vi "OPC.vi"(8 "error in (no error)":errorcluster, 11 "E5071C in":refnum<class "E5071C.lvclass">) -> (0 "error out":errorcluster, 3 "E5071C out":refnum<class "E5071C.lvclass">)   [LabVIEW 2020, in "E5071C.lvlib" / "E5071C.lvclass"]
uses:
  E5071C.lvclass
  E5071C.lvclass/E5071C.ctl
panel:
  out "String":string
  in  "Number Of Bytes":i32=-1
  out "Returned Bytes":i32
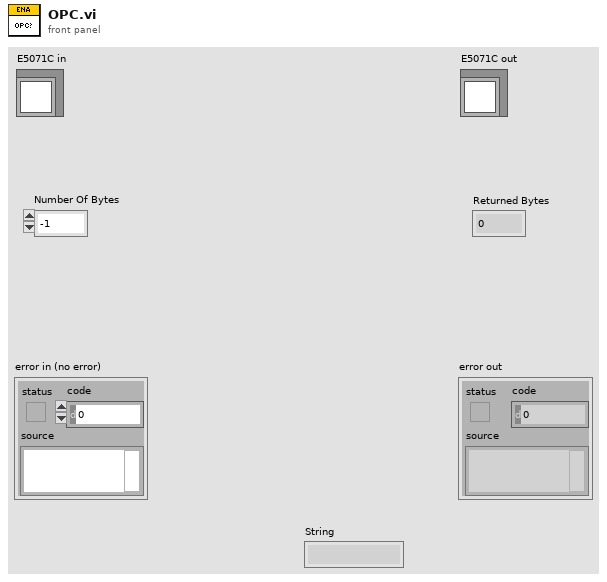
[diagram p1: front panel]
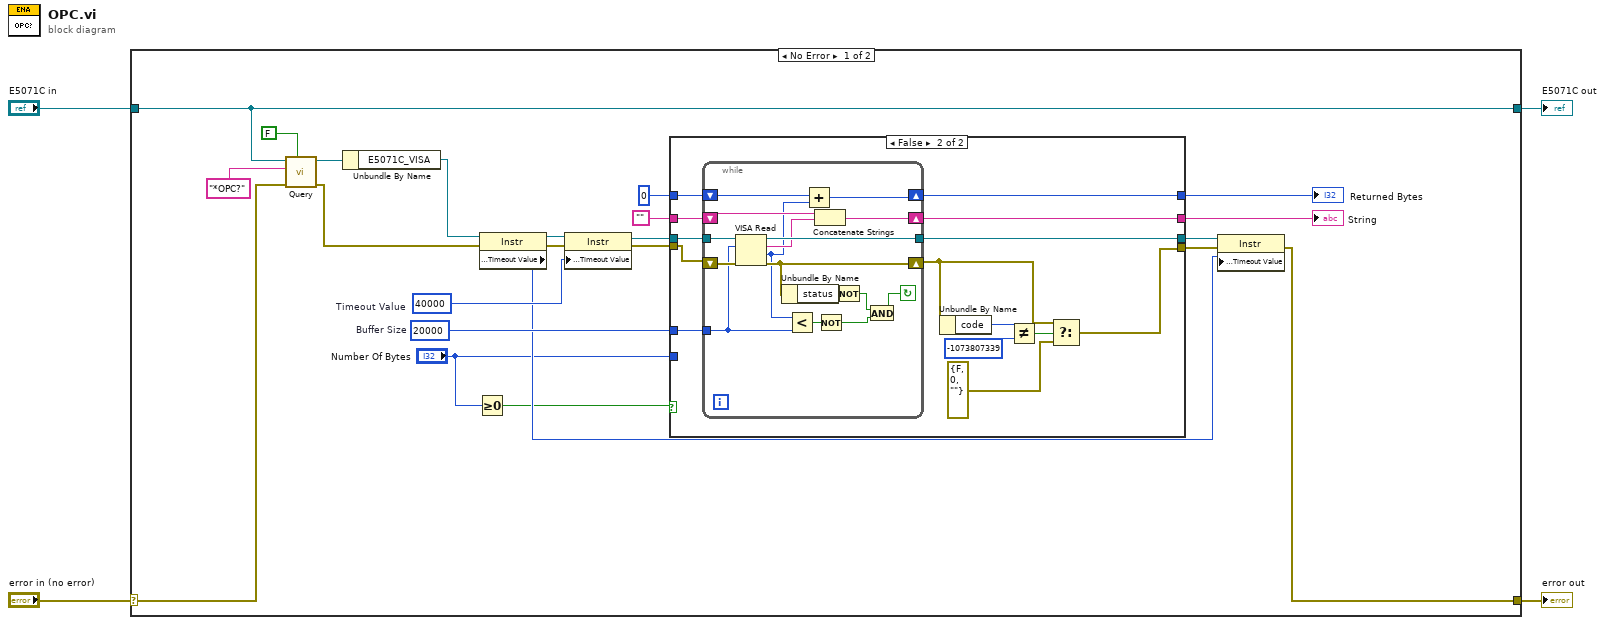
[diagram p0: block diagram]
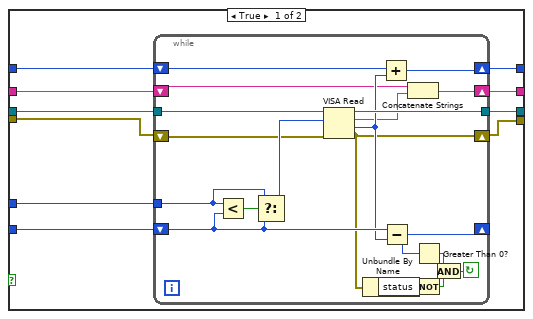
[diagram p2: hidden frame]
diagram:
  n1 = case shown="No Error" "error in (no error)" {
    selector: "error in (no error)" -> [w24 w88]
    tunnel: [w5 w88] -> w3
    tunnel: [w27 w87] -> w1
    tunnel: "E5071C in" -> [w27 w87]
    frame No Error {
      w15 = u32 40000  # Timeout Value
      w20 = u32 20000  # Buffer Size
      n2 = call "Query.vi"("Return"=FALSE, "error in (no error)"=w24, "Command"="*OPC?" ("write buffer"), "E5071C in"=w27) -> ("error out"=w6:errorcluster, "E5071C out"=w23:refnum<class "E5071C.lvclass">)  [unwired: 5 in, 1 out]
      n3 = Unbundle By Name(w23) -> ("E5071C_VISA"=w7:refnum<visa-resource-name>)
      n4 = Greater Or Equal To 0?(x="Number Of Bytes") -> (x >= 0?=w8:bool)
      n5 = property class="Instr"(reference=w7, error in=w6) -> (reference out=w17:refnum<visa-resource-name>, error out=w16:errorcluster, "General Settings:Timeout Value"=w10:u32)
      n6 = property class="Instr"(reference=w17, error in=w16, "General Settings:Timeout Value"=w15) -> (reference out=w13:refnum<visa-resource-name>, error out=w14:errorcluster)
      n7 = case shown="False" w8 {
        tunnel: "" -> [w37 w70]
        tunnel: [w36 w69] -> w21
        tunnel: w20 -> [w35 w68]
        tunnel: "Number Of Bytes" -> [w34 _]
        tunnel: u32 0 ("byte count (0)") -> [w33 w67]
        tunnel: [w32 w66] -> w18
        tunnel: w14 -> [w31 w65]
        tunnel: w13 -> [w30 w64]
        tunnel: [w29 w63] -> w12
        tunnel: [w28 w57] -> w11
        frame True {
          n8 = while {
            shift-left: w37 -> [w41]
            shift-right: [w42] -> w32
            tunnel: w35 -> [w50]
            shift-left: w33 -> [w48]
            shift-right: [w47] -> w36
            shift-left: w34 -> [w52]
            shift-right: [w51] -> _
            shift-left: w31 -> [w38]
            shift-right: [w39] -> w28
            tunnel: [w55] -> w29
            tunnel: w30 -> [w56]
            stop <- w43 continue-if-true
            n9 = Less?(x=w50, y=w52) -> (x < y?=w54:bool)
            n10 = Select(t=w50, s=w54, f=w52) -> (s? t:f=w53:u32)
            n11 = VISA Read(VISA resource name=w56, byte count=w53, error in (no error)=w38) -> (VISA resource name out=w55:refnum<visa-resource-name>, read buffer=w40:string, return count=w49:u32, error out=w39:errorcluster)
            n12 = Unbundle By Name(w39) -> ("status"=w45:bool)
            n13 = Add(x=w48, y=w49) -> (x+y=w47:u32)
            n14 = Subtract(x=w52, y=w49) -> (x-y=w51:u32)
            n15 = Concatenate Strings(w41, w40) -> (w42:string)
            n16 = Greater Than 0?(x=w51) -> (x > 0?=w46:bool)
            n17 = Not(x=w45) -> (.not. x?=w44:bool)
            n18 = And(x=w46, y=w44) -> (x .and. y?=w43:bool)
          }
        }
        frame False {
          n19 = while {
            shift-left: w70 -> [w80]
            shift-right: [w81] -> w66
            tunnel: w68 -> [w71]
            shift-left: w67 -> [w84]
            shift-right: [w83] -> w69
            shift-left: w65 -> [w77]
            shift-right: [w78] -> w59
            tunnel: [w85] -> w63
            tunnel: w64 -> [w86]
            stop <- w73 continue-if-true
            n20 = VISA Read(VISA resource name=w86, byte count=w71, error in (no error)=w77) -> (VISA resource name out=w85:refnum<visa-resource-name>, read buffer=w79:string, return count=w72:u32, error out=w78:errorcluster)
            n21 = Unbundle By Name(w78) -> ("status"=w82:bool)
            n22 = Less?(x=w72, y=w71) -> (x < y?=w76:bool)
            n23 = Add(x=w84, y=w72) -> (x+y=w83:u32)
            n24 = Concatenate Strings(w80, w79) -> (w81:string)
            n25 = Not(x=w76) -> (.not. x?=w75:bool)
            n26 = Not(x=w82) -> (.not. x?=w74:bool)
            n27 = And(x=w74, y=w75) -> (x .and. y?=w73:bool)
          }
          n28 = Unbundle By Name(w59) -> ("code"=w62:i32)
          n29 = Not Equal?(x=w62, y=-1073807339) -> (x != y?=w60:bool)
          n30 = Select(t=w59, s=w60, f=errorcluster {"status"=FALSE, "code"=0, "source"=""}) -> (s? t:f=w57:errorcluster)
        }
      }
      "Returned Bytes" <- w21
      "String" <- w18
      n31 = property class="Instr"(reference=w12, error in=w11, "General Settings:Timeout Value"=w10) -> (error out=w5:errorcluster)  [unwired: 1 out]
    }
    frame Error {
    }
  }
  "error out" <- w3
  "E5071C out" <- w1
